vi "Shutdown - flush.vi"(8 "error in (no error)":errorcluster) -> (0 "error out":errorcluster)   [LabVIEW 2026, in "Tests.lvlib"]
doc: "Verifies SRS-LMBR-002: statements logged before shutdown are flushed to the sink before Logger.Shutdown returns (the flush fence). Logs a burst to a file appender, calls Shutdown, then asserts every statement is present in the file in order, so none were lost to a premature stop.\n\nImplements LMBR-T-052 -> SRS-002. Assert-level IDs: Test-ID-Assert-Checklist.md."
uses:
  Tests.lvlib
  src/TypeDefs/Severity.ctl
  src/TypeDefs/FileAppenderConfig.ctl
  src/TypeDefs/AppenderConfig.ctl
  src/TypeDefs/Filter.ctl
  src/TypeDefs/FilterMode.ctl
  src/TypeDefs/DropPolicy.ctl
  src/TypeDefs/FileConfig.ctl
  <vilib>/addons/_JKI Toolkits/Caraya/classes/Assert/Assert Equal Value_Variant.vi
  <vilib>/addons/_JKI Toolkits/Caraya/classes/Assert/Assert True.vi
  <vilib>/addons/_JKI Toolkits/Caraya/classes/Test/Test.lvclass
  src/Lumberjack.lvlib
  src/Public/Logger.lvclass/Logger.lvclass
  <vilib>/addons/_JKI Toolkits/Caraya/classes/Assert/Assert.lvclass
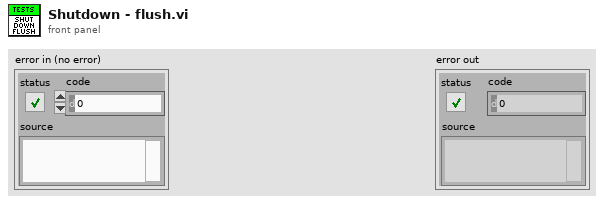
[diagram p1: front panel]
types:
  T1 = typedef "Lumberjack.lvlib/Severity.ctl" = enum16{"OFF", "FATAL", "ERROR", "WARN", "INFO", "DEBUG", "TRACE", "ALL"}
  T2 = typedef "Lumberjack.lvlib/FileAppenderConfig.ctl" = cluster{"common":T3, "file":T7}
  T3 = typedef "Lumberjack.lvlib/AppenderConfig.ctl" = cluster{"id":string, "threshold":T1, "filter":T4, "queueBound":i32, "dropPolicy":T6, "useUTC":bool}
  T4 = typedef "Lumberjack.lvlib/Filter.ctl" = cluster{"mode":T5, "levelMin":T1, "levelMax":T1, "tagPrefix":string}
  T5 = typedef "Lumberjack.lvlib/FilterMode.ctl" = enum16{"Mirror", "Routed"}
  T6 = typedef "Lumberjack.lvlib/DropPolicy.ctl" = enum16{"DropOldest", "DropNewest", "LevelAware"}
  T7 = typedef "Lumberjack.lvlib/FileConfig.ctl" = cluster{"rootFolder":path, "maxFileSize":i64, "maxFileCount":i32, "baseName":string, "extension":string, "delimiter":string, "calendarFolderTree":bool}
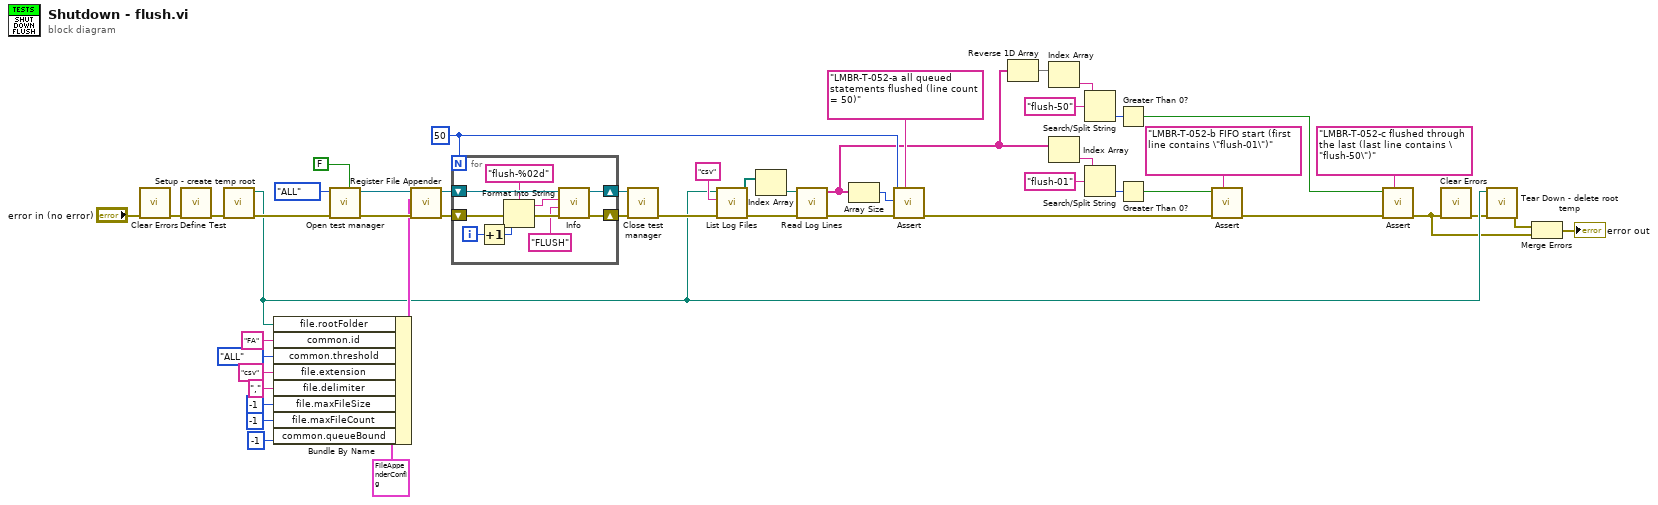
[diagram p0: block diagram]
diagram:
  w17 = 50
  n1 = call <vilib>:"Clear Errors.vi"("error in (no error)"="error in (no error)") -> ("error out"=w23:errorcluster)  [unwired: 5 in, 1 out]
  n2 = call <vilib>:"Define Test.vi"("error in (no error)"=w23) -> ("error out"=w48:errorcluster)  [unwired: 9 in, 1 out]
  n3 = call "Setup - create temp root.vi"("error in (no error)"=w48) -> ("error out"=w28:errorcluster, "tempRoot"=w3:path)  [unwired: 9 in]
  n4 = Bundle By Name(cluster=T2 {"common"={"id"="", "threshold"=enum."INFO", "filter"={"mode"=enum."Mirror", "levelMin"=enum."INFO", "levelMax"=enum."INFO", "tagPrefix"=""}, "queueBound"=0, "dropPolicy"=enum."DropOldest", "useUTC"=FALSE}, "file"={"rootFolder"=path "", "maxFileSize"=0, "maxFileCount"=0, "baseName"="", "extension"="", "delimiter"="", "calendarFolderTree"=FALSE}} ("FileAppenderConfig"), "file.rootFolder"=w3, "common.id"="FA", "common.threshold"=Severity."ALL", "file.extension"="csv", "file.delimiter"=",", "file.maxFileSize"=i64 -1, "file.maxFileCount"=-1, "common.queueBound"=-1) -> (w42:T2)
  n5 = call "Open test manager.vi"("enableDefaultFile"=FALSE, "error in (no error)"=w28, "globalThreshold"=Severity."ALL") -> ("error out"=w46:errorcluster, "Logger out"=w41:refnum<class "Logger.lvclass">)  [unwired: 7 in]
  n6 = call "Register File Appender.vi"("error in (no error)"=w46, "FileAppenderConfig"=w42, "Logger in"=w41) -> ("error out"=w45:errorcluster, "Logger out"=w40:refnum<class "Logger.lvclass">)  [unwired: 6 in, 1 out]
  n7 = for {
    N: w17 -> [_]
    shift-right: [w58] -> w38
    shift-left: w45 -> [w56]
    shift-right: [w57] -> w37
    shift-left: w40 -> [w59]
    i -> [w53]
    n8 = Increment(x=w53) -> (x+1=w52:i32)
    n9 = Format Into String(format string="flush-%02d" ("sourceTag"), error in=w56, w52) -> (resulting string=w51:string, error out=w55:errorcluster)  [unwired: 1 in]
    n10 = call "Info.vi"("error in (no error)"=w55, "sourceTag"="FLUSH", "message"=w51, "Logger in"=w59) -> ("error out"=w58:errorcluster, "Logger out"=w57:refnum<class "Logger.lvclass">)  [unwired: 6 in]
  }
  n11 = call "Close test manager.vi"("error in (no error)"=w38, "Logger in"=w37) -> ("error out"=w26:errorcluster)  [unwired: 7 in]
  n12 = call "List Log Files.vi"("error in (no error)"=w26, "extension"="csv", "rootFolder"=w3) -> ("error out"=w22:errorcluster, "filePaths"=w36:path[])  [unwired: 6 in, 1 out]
  n13 = Index Array(array=w36) -> (element=w25:path)  [unwired: 1 in]
  n14 = call "Read Log Lines.vi"("error in (no error)"=w22, "filePath"=w25) -> ("error out"=w20:errorcluster, "lines"=w11:string[])  [unwired: 8 in]
  n15 = Array Size(array=w11) -> (size(s)=w18:i32)
  n16 = call-poly <vilib>:"Assert.vi"("Label"="LMBR-T-052-a all queued statements flushed (line count = 50)", "error in (no error)"=w20, "Actual"=w18, "Expected"=w17) -> ("error out"=w19:errorcluster)  [unwired: 6 in, 1 out]
  n17 = Reverse 1D Array(array=w11) -> (reversed array=w10:string[])
  n18 = Index Array(array=w10) -> (element=w14:string)  [unwired: 1 in]
  n19 = Index Array(array=w11) -> (element=w29:string)  [unwired: 1 in]
  n20 = Search/Split String(string=w14, search string/char (-)="flush-50") -> (offset of match=w9:i32)  [unwired: 1 in, 2 out]
  n21 = Search/Split String(string=w29, search string/char (-)="flush-01") -> (offset of match=w35:i32)  [unwired: 1 in, 2 out]
  n22 = Greater Than 0?(x=w9) -> (x > 0?=w8:bool)
  n23 = Greater Than 0?(x=w35) -> (x > 0?=w34:bool)
  n24 = call-poly <vilib>:"Assert.vi"("Label"="LMBR-T-052-b FIFO start (first line contains \"flush-01\")", "error in (no error)"=w19, "True?"=w34) -> ("error out"=w7:errorcluster)  [unwired: 7 in, 1 out]
  n25 = call-poly <vilib>:"Assert.vi"("Label"="LMBR-T-052-c flushed through the last (last line contains \"flush-50\")", "error in (no error)"=w7, "True?"=w8) -> ("error out"=w2:errorcluster)  [unwired: 7 in, 1 out]
  n26 = call <vilib>:"Clear Errors.vi"("error in (no error)"=w2) -> ("error out"=w1:errorcluster)  [unwired: 5 in, 1 out]
  n27 = call "Tear Down - delete root temp.vi"("error in (no error)"=w1, "tempRoot"=w3) -> ("error out"=w5:errorcluster)  [unwired: 9 in]
  n28 = Merge Errors(w5, w2) -> (→"error out":errorcluster)
